vi "Alignment.vi"() -> ()   [LabVIEW 2010]
uses:
  <vilib>/Utility/inputDevices.llb/closeKeyboard.vi
  <vilib>/Utility/inputDevices.llb/keyboardAcquire.vi
panel:
  out "keys pressed":T1(array[ring])
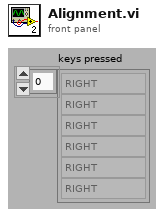
[diagram p1: front panel]
types:
  T1 = enum16{"0", "1", "2", "3", "4", "5", "6", "7", "8", "9", "A", "B", "C", "D", "E", "F", "G", "H", "I", "J", "K", "L", "M", "N", "O", "P", "Q", "R", "S", "T", "U", "V", "W", "X", "Y", "Z", "F1", "F2", "F3", "F4", "F5", "F6", "F7", "F8", "F9", "F10", "F11", "F12", "F13", "F14", "F15", "ADD", "BACK", "BACKSLASH", "CAPITAL", "COMMA", "DECIMAL", "DELETE", "DIVIDE", "DOWN", "END", "EQUALS", "ESCAPE", "GRAVE (`)", "HOME", "INSERT", "LBRACKET", "LCONTROL", "LEFT", "L ALT", "LSHIFT", "LWIN", "MINUS", "MULTIPLY", "NEXT", "NUMLOCK", "NUMPAD_0", "NUMPAD_1", "NUMPAD_2", "NUMPAD_3", "NUMPAD_4", "NUMPAD_5", "NUMPAD_6", "NUMPAD_7", "NUMPAD_8", "NUMPAD_9", "PAUSE", "PERIOD", "PRIOR (PG UP)", "RBRACKET", "RCONTROL", "RETURN", "RIGHT", "R ALT", "RSHIFT", "RWIN", "SCROLL", "SEMICOLON", "SLASH", "SPACE", "SUBTRACT", "TAB", "UP", "ENTER (num pad)", "' (quote)"}[]
  T2 = enum16{"0", "1", "2", "3", "4", "5", "6", "7", "8", "9", "A", "B", "C", "D", "E", "F", "G", "H", "I", "J", "K", "L", "M", "N", "O", "P", "Q", "R", "S", "T", "U", "V", "W", "X", "Y", "Z", "F1", "F2", "F3", "F4", "F5", "F6", "F7", "F8", "F9", "F10", "F11", "F12", "F13", "F14", "F15", "ADD", "BACK", "BACKSLASH", "CAPITAL", "COMMA", "DECIMAL", "DELETE", "DIVIDE", "DOWN", "END", "EQUALS", "ESCAPE", "GRAVE (`)", "HOME", "INSERT", "LBRACKET", "LCONTROL", "LEFT", "L ALT", "LSHIFT", "LWIN", "MINUS", "MULTIPLY", "NEXT", "NUMLOCK", "NUMPAD_0", "NUMPAD_1", "NUMPAD_2", "NUMPAD_3", "NUMPAD_4", "NUMPAD_5", "NUMPAD_6", "NUMPAD_7", "NUMPAD_8", "NUMPAD_9", "PAUSE", "PERIOD", "PRIOR (PG UP)", "RBRACKET", "RCONTROL", "RETURN", "RIGHT", "R ALT", "RSHIFT", "RWIN", "SCROLL", "SEMICOLON", "SLASH", "SPACE", "SUBTRACT", "TAB", "UP", "ENTER (num pad)", "' (quote)"}
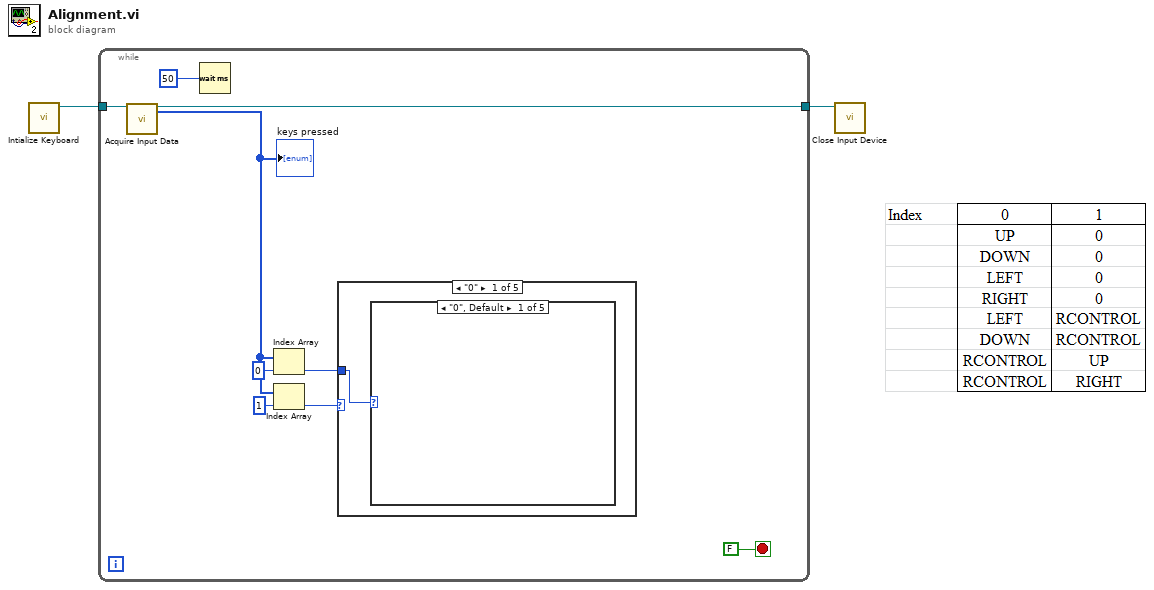
[diagram p0: block diagram]
diagram:
  n1 = call <vilib>:"Intialize Keyboard.vi"() -> ("device ID"=w1:refnum<k1>)  [unwired: 10 in, 1 out]
  n2 = while {
    tunnel: w1 -> [w11]
    tunnel: [w10] -> w2
    stop <- FALSE stop-if-true
    n3 = call-poly <vilib>:"Acquire Input Data.vi"("device ID"=w11) -> ("device ID"=w10:refnum<k1>, "keys pressed"=w7:T1)  [unwired: 16 in, 1 out]
    "keys pressed" <- w7
    n4 = Wait (ms)(milliseconds to wait=50 ("timeout ms (-1 never timeout)")) -> ()  [unwired: 1 out]
    n5 = Index Array(array=w7, index=0) -> (element=w3:T2)
    n6 = Index Array(array=w7, index=1) -> (element=w4:T2)
    n7 = case shown="\"0\"" w4 {
      tunnel: w3 -> [w12 w13 w14 w15 _]
      frame "0" {
        n8 = case shown="\"0\", Default" w12 {
          frame "0", Default {
          }
          frame "UP" {
          }
          frame "DOWN" {
          }
          frame "LEFT" {
          }
          frame "RIGHT" {
          }
        }
      }
      frame "UP" {
        n9 = case shown="\"2\", Default" w13 {
          frame "RCONTROL" {
          }
          frame "2", Default {
          }
        }
      }
      frame "RIGHT" {
        n10 = case shown="\"RCONTROL\"" w14 {
          frame "RCONTROL" {
          }
          frame "2", Default {
          }
        }
      }
      frame "RCONTROL" {
        n11 = case shown="\"LEFT\"" w15 {
          frame "0", Default {
          }
          frame "LEFT" {
          }
          frame "DOWN" {
          }
        }
      }
      frame "2", Default {
      }
    }
  }
  n12 = call-poly <vilib>:"Close Input Device.vi"("device ID"=w2) -> ()  [unwired: 9 in, 1 out]
